vi "SAI_panel_codigo.vi"() -> ()   [LabVIEW 2024, in "SALICRU_MODBUS.lvlib"]
uses:
  <vilib>/Modbus/master/Create Master Instance (TCP).vi
  <vilib>/Modbus/master/Modbus Master.lvclass
  SALICRU_MODBUS.lvlib
panel:
  out "salida Vt":dbl
  out "salida Vs":dbl
  out "salida Vr":dbl
  out "Porcentaje P":dbl
  out "corrinte T":dbl format="%.2f"
  out "corriente S":dbl format="%.2f"
  out "corriente R":dbl format="%.2f"
  out "Tin":u16
  out "Sin":u16
  out "Rin":u16
  out "bypass(F), line (T)":bool
  out "Work mode":string
  in  "stop 2":bool
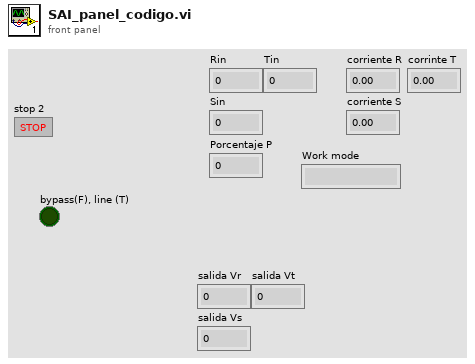
[diagram p1: front panel]
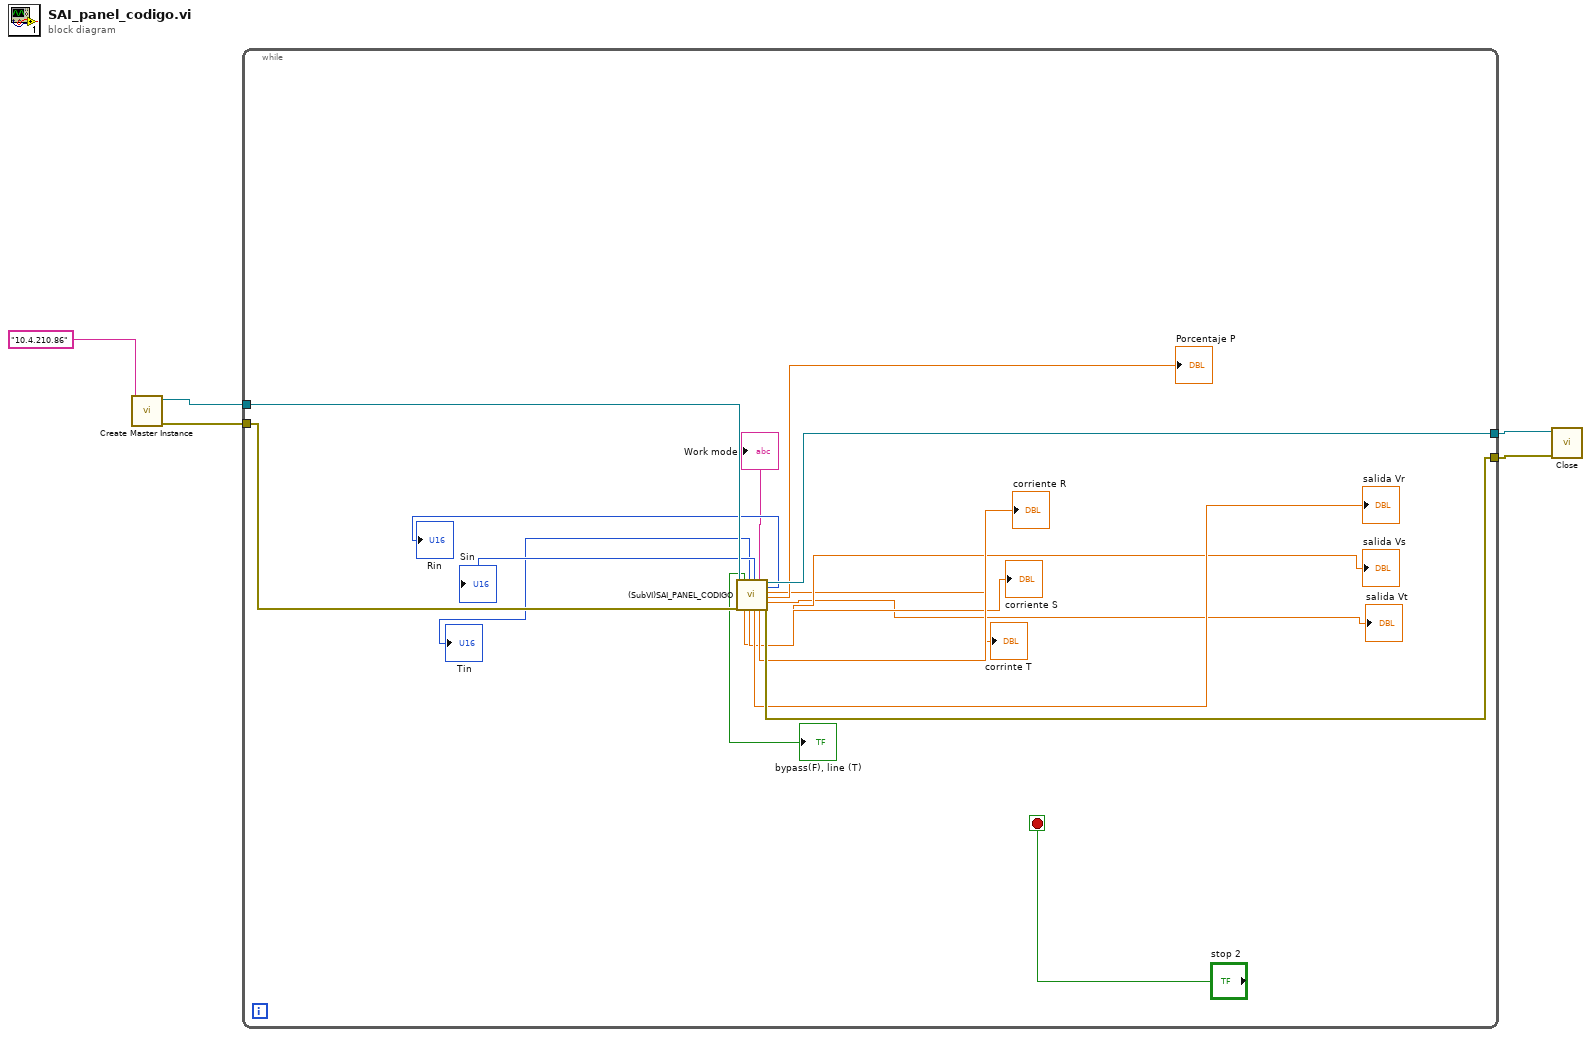
[diagram p0: block diagram]
diagram:
  n1 = call-poly <vilib>:"Create Master Instance.vi"("address"="10.4.210.86") -> ("error out"=w3:errorcluster, "TCP master instance"=w4:refnum<class "Modbus Master.lvclass">)  [unwired: 9 in]
  n2 = while {
    tunnel: w4 -> [w21]
    tunnel: w3 -> [w20]
    tunnel: [w19] -> w2
    tunnel: [w18] -> w1
    stop <- "stop 2" stop-if-true
    n3 = call "(SubVI)SAI_PANEL_CODIGO.vi"("Modbus Master in"=w21, "error in (no error)"=w20) -> ("bypass(F), line (T)"=→"bypass(F), line (T)":bool, "salida Vs"=→"salida Vs":dbl, "Tin"=→"Tin":u16, "corriente S"=→"corriente S":dbl, "Sin"=→"Sin":u16, "salida Vr"=→"salida Vr":dbl, "Work mode"=→"Work mode":string, "corriente R"=→"corriente R":dbl, "Modbus Master out"=w18:refnum<class "Modbus Master.lvclass">, "Rin"=→"Rin":u16, "corrinte T"=→"corrinte T":dbl, "Porcentaje P"=→"Porcentaje P":dbl, "salida Vt"=→"salida Vt":dbl, "error out"=w19:errorcluster)  [unwired: 4 in]
  }
  n4 = call-dynamic "Close.vi"("error in (no error)"=w2, "Modbus master in"=w1) -> ()  [unwired: 9 in, 1 out]
